vi "cam.vi"() -> ()   [LabVIEW 2015]
uses:
  <vilib>/userdefined/High Color/IMAQdx.ctl
  <vilib>/vision/driver/NI_Vision_Acquisition_Software.lvlib
panel:
  out "error out":errorcluster
  in  "Take image":bool=TRUE
  in  "Stop Camera":bool=TRUE
  in  "Start Camera":bool=TRUE
  in  "Session In":T1
  out "Image":T2(plugin-control)
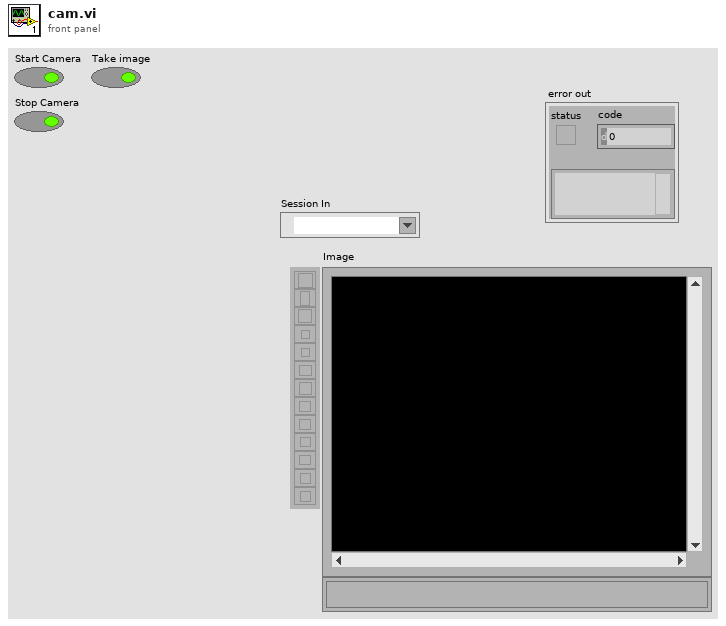
[diagram p1: front panel]
types:
  T1 = typedef "IMAQdx.ctl" = refnum<k21>
  T2 = typedef "IMAQ Image.ctl" = refnum<image>
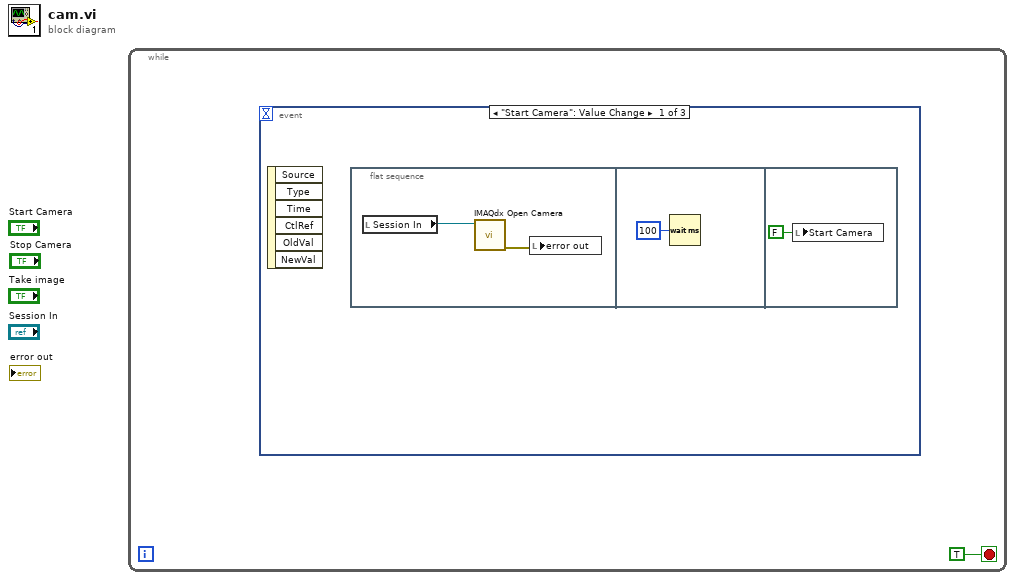
[diagram p0: block diagram]
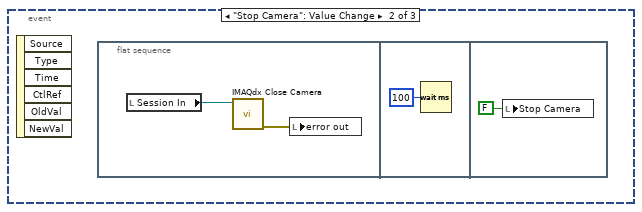
[diagram p2: hidden frame]
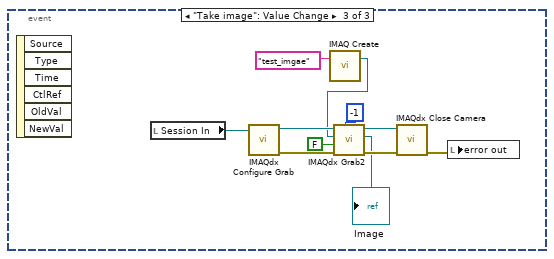
[diagram p3: hidden frame]
diagram:
  n1 = while {
    stop <- TRUE stop-if-true
    n2 = event shown="[0] \"Start Camera\": Value Change" {
      selector: _ -> [_ _ _]
      dyn-events: _ -> [_ _ _]
      timeout: _ -> [_ _ _]
      event "Start Camera": Value Change {
        n3 = event-data() -> ()  [unwired: 1 in, 6 out]
        n4 = flat-sequence {
          frame #0 {
            n5 = local read "Session In"() -> (w3:T1)
            n6 = call <vilib>:"IMAQdx Open Camera.vi"("Session In"=w3) -> ("error out"=w2:errorcluster)  [unwired: 9 in, 1 out]
            n7 = local write "error out"(w2) -> ()
          }
          frame #1 {
            n8 = Wait (ms)(milliseconds to wait=u32 100) -> ()  [unwired: 1 out]
          }
          frame #2 {
            n9 = local write "Start Camera"(FALSE ("Start Camera")) -> ()
          }
        }
      }
      event "Stop Camera": Value Change {
        n10 = event-data() -> ()  [unwired: 1 in, 6 out]
        n11 = flat-sequence {
          frame #0 {
            n12 = local read "Session In"() -> (w7:T1)
            n13 = call <vilib>:"IMAQdx Close Camera.vi"("Session In"=w7) -> ("error out"=w6:errorcluster)  [unwired: 10 in]
            n14 = local write "error out"(w6) -> ()
          }
          frame #1 {
            n15 = Wait (ms)(milliseconds to wait=u32 100 ("millisecond timer value")) -> ()  [unwired: 1 out]
          }
          frame #2 {
            n16 = local write "Stop Camera"(FALSE ("Stop Camera")) -> ()
          }
        }
      }
      event "Take image": Value Change {
        n17 = event-data() -> ()  [unwired: 1 in, 6 out]
        n18 = local read "Session In"() -> (w11:T1)
        n19 = call <vilib>:"IMAQdx Configure Grab.vi"("Session In"=w11) -> ("error out"=w14:errorcluster, "Session Out"=w20:T1)  [unwired: 9 in]
        n20 = call "IMAQ Create"("Image Name"="test_imgae") -> ("New Image"=w16:T2)  [unwired: 4 in, 1 out]
        n21 = call <vilib>:"IMAQdx Grab2.vi"("Timeout (ms)"=-1, "error in"=w14, "Wait for Next Buffer? (Yes)"=FALSE, "Image In"=w16, "Session In"=w20) -> ("error out"=w19:errorcluster, "Image Out"=→"Image":T2, "Session Out"=w18:T1)  [unwired: 3 in, 1 out]
        n22 = call <vilib>:"IMAQdx Close Camera.vi"("error in"=w19, "Session In"=w18) -> ("error out"=w10:errorcluster)  [unwired: 9 in]
        n23 = local write "error out"(w10) -> ()
      }
    }
  }
